vi "S7COMM - Parse Response - Decode Read Item - Split Data Array.vi"(8 "error in (no error)":errorcluster, 11 "Response Data IN":T1 format="0x%02x") -> (0 "error out":errorcluster, 1 "Transport Data Type":T3=4 items=["Single Bit [bits]"=3, "Bit Octets [bits]"=4, "Bit Double Octets [bits]"=5, "Real [bytes]"=7, "Char [bytes]"=9], 2 "Count":u16, 3 "Rest of Response Data":T1 format="0x%02x")   [LabVIEW 2014, in "S7NetCom.lvclass"]
doc: "____\nCopyright (c) 2019 Hampel Software Engineering (HSE), released under BSD license. More info can be found on https://dokuwiki.hampel-soft.com/code/hse/s7netcom. Original code published by Marc Christenson, Sisu Devices."
uses:
  S7NetCom.lvclass
  Controls/S7NetCom_HexByteArray.ctl
  Controls/S7NetCom_HexByte.ctl
  S7COMM - Transport Data Types--ring.ctl
  S7COMM - Response Item Return Code-error.vi
panel:
  # "More info on https://dokuwiki.hampel-soft.com/code/hse/s7netcom\n\nCopyright (c) 2019, HAMPEL SOFTWARE ENGINEERING (HSE)\nOriginal code developed by Marc Christenson, Sisu Devices\nAll rights reserved.\n\nRedistribution and use in source and binary forms, with or without\nmodification, are permitted provided that the following conditions are met:\n\n1. Redistributions of source code must retain the above copyright\n   notice, this list of conditions and the following disclaimer.\n\n2. Redistributions in binary form must reproduce the above copyright\n   notice, this list of conditions and the following disclaimer in the\n   documentation and/or other materials provided with the distribution.\n\n3. All advertising materials mentioning features or use of this software\n   must display the following acknowledgement:\n   This product includes software developed by HAMPEL SOFTWARE ENGINEERING.\n\n4. Neither the name of HAMPEL SOFTWARE ENGINEERING nor the\n   names of its contributors may be used to endorse or promote products\n   derived from this software without specific prior written permission.\n\nTHIS SOFTWARE IS PROVIDED BY HAMPEL SOFTWARE ENGINEERING ''AS IS'' AND ANY\nEXPRESS OR IMPLIED WARRANTIES, INCLUDING, BUT NOT LIMITED TO, THE IMPLIED\nWARRANTIES OF MERCHANTABILITY AND FITNESS FOR A PARTICULAR PURPOSE ARE\nDISCLAIMED. IN NO EVENT SHALL HAMPEL SOFTWARE ENGINEERING BE LIABLE FOR ANY\nDIRECT, INDIRECT, INCIDENTAL, SPECIAL, EXEMPLARY, OR CONSEQUENTIAL DAMAGES\n(INCLUDING, BUT NOT LIMITED TO, PROCUREMENT OF SUBSTITUTE GOODS OR SERVICES;\nLOSS OF USE, DATA, OR PROFITS; OR BUSINESS INTERRUPTION) HOWEVER CAUSED AND\nON ANY THEORY OF LIABILITY, WHETHER IN CONTRACT, STRICT LIABILITY, OR TORT\n(INCLUDING NEGLIGENCE OR OTHERWISE) ARISING IN ANY WAY OUT OF THE USE OF THIS\nSOFTWARE, EVEN IF ADVISED OF THE POSSIBILITY OF SUCH DAMAGE."
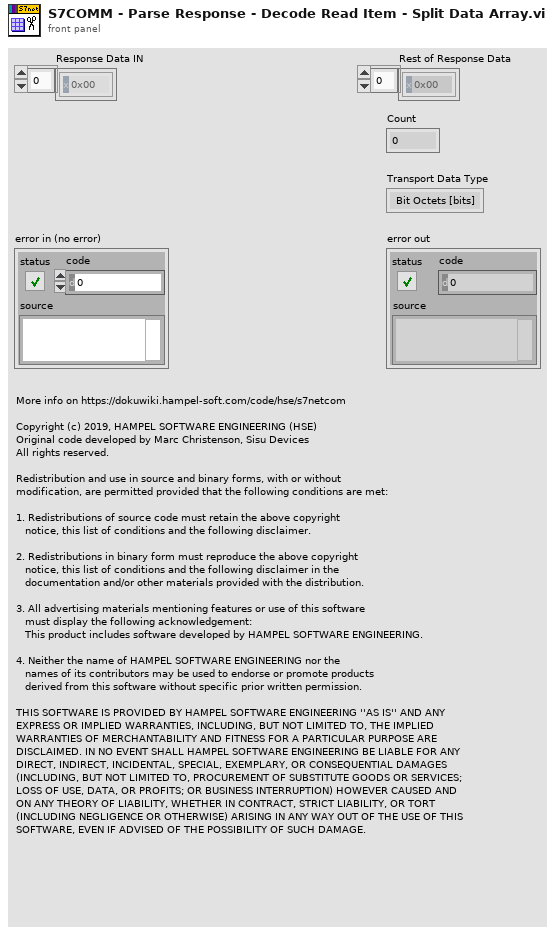
[diagram p1: front panel]
types:
  T1 = typedef "S7NetCom.lvclass/S7NetCom_HexByteArray.ctl" = T2[]
  T2 = typedef "S7NetCom.lvclass/S7NetCom_HexByte.ctl" = u8
  T3 = typedef "S7NetCom.lvclass/S7COMM - Transport Data Types--ring.ctl" = u8
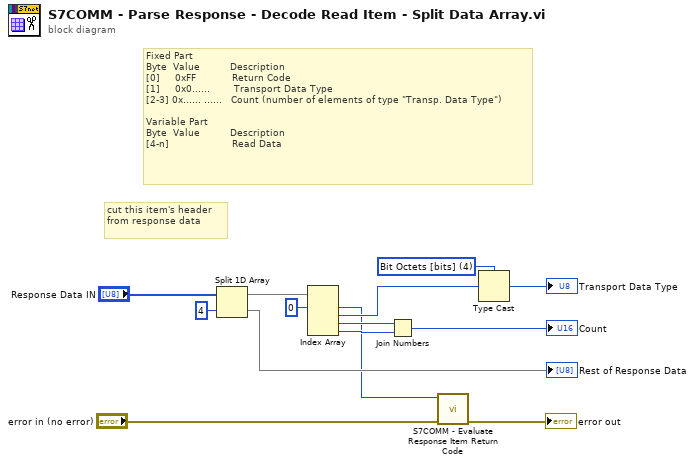
[diagram p0: block diagram]
diagram:
  w6 = T3 4 items=["Single Bit [bits]"=3, "Bit Octets [bits]"=4, "Bit Double Octets [bits]"=5, "Real [bytes]"=7, "Char [bytes]"=9] ("Reply Data Types")
  # "cut this item's header from response data"
  # "Fixed Part\nByte\t Value\t         Description\n[0]\t    0xFF\t           Return Code\n[1]\t    0x0……\t       Transport Data Type\n[2-3]\t0x…… ……\t  Count (number of elements of type \"Transp. Data Type\")\n\nVariable Part\nByte\t Value\t         Description\n[4-n]\t\t                   Read Data"
  n1 = Split 1D Array(array="Response Data IN", index=4) -> (first subarray=w12:T1, second subarray=→"Rest of Response Data":T1)
  n2 = Index Array(array=w12, index #1=0) -> (element #1=w1:T2, element #2=w5:T2, element #3=w9:T2, element #4=w10:T2)  [unwired: 3 in]
  n3 = Join Numbers(hi=w9, lo=w10) -> ((hi.lo)=→"Count":u16)
  n4 = call "S7COMM - Evaluate Response Item Return Code.vi"("error in (no error)"="error in (no error)", "Return Code"=w1) -> ("error out"=→"error out":errorcluster)  [unwired: 9 in]
  n5 = Type Cast(type=w6, x=w5) -> (*(type *) &x=→"Transport Data Type":T3)
